vi "test_DataCollectionDL090215.vi"() -> ()   [LabVIEW 2010, in "DataCollectionDL090215.lvclass"]
uses:
  DataCollectionDL090215.lvclass
  common/classes/Image/Image/Image.lvclass
  main/labview_source/type_definitions/clusters/controls_refs.ctl
  common/classes/ErrorController/ErrorController/ErrorController.lvclass
  GenericDataCollection/GenericDataCollection/trigger_enum.ctl
  GenericDataCollection/GenericDataCollection/GenericDataCollection.lvclass
  common/classes/GenericToplevelComponent/GenericToplevelComponent/common_trigger_enum.ctl
  common/classes/GenericToplevelComponent/GenericToplevelComponent/GenericToplevelComponent.lvclass
panel:
  in  "images per sweep":i32
  in  "create":bool
  in  "reset":bool
  in  "save":bool
  out "event handling loop counter":i32=5
  in  "image index":i32
  in  "sweep index":i32
  in  "update":bool
  in  "retrieve":bool
  in  "insert":bool
  in  "stop":bool
  # "Test DL090215DataCollection"
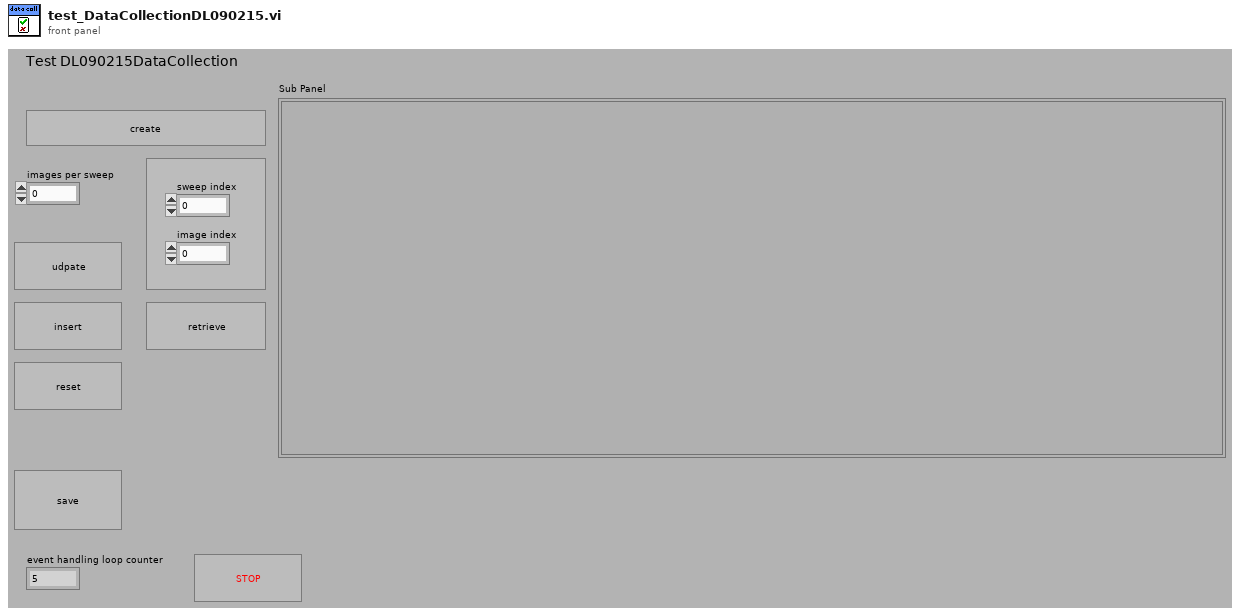
[diagram p1: front panel]
types:
  T1 = typedef "controls_refs.ctl" = cluster{"scan start button":refnum<vi>, "tabs":cluster{"main":refnum<vi>, "settings":refnum<vi>}, "subpanels":cluster{"imagingMode":refnum<vi>, "scanHead":refnum<vi>, "display":refnum<vi>, "experimentController":refnum<vi>, "instrument":refnum<vi>, "stage":refnum<vi>, "stimulator":refnum<vi>, "dataCollection":refnum<vi>, "analyser":refnum<vi>, "daq":refnum<vi>, "imageAssembler":refnum<vi>}, "drop-downs":cluster{"run mode":refnum<vi>, "imagingMode":refnum<vi>, "experimentalController":refnum<vi>, "objective":refnum<vi>}, "status lights":cluster{"experimentController":refnum<vi>, "imagingMode":refnum<vi>, "scanHead":refnum<vi>, "daq":refnum<vi>, "imageAssembler":refnum<vi>, "dataCollection":refnum<vi>, "display":refnum<vi>, "analyser":refnum<vi>, "stage":refnum<vi>, "stimulator":refnum<vi>, "instrument":refnum<vi>}, "message":refnum<vi>, "stimulator enabled?":refnum<vi>, "saving":cluster{"data folder path":refnum<vi>, "file base name":refnum<vi>, "notebook":refnum<vi>}, "progress bar":refnum<vi>, "update icon":refnum<vi>, "title":refnum<vi>, "main vi":refnum<vi>, "user":refnum<vi>, "exit_button":refnum<vi>, "CPU usage %":refnum<vi>}
  T2 = typedef "GenericDataCollection.lvclass/trigger_enum.ctl" = enum16{"NULL", "save"}
  T3 = typedef "GenericToplevelComponent.lvclass/common_trigger_enum.ctl" = enum16{"NULL", "initialise", "terminate", "fetch command", "fetch data", "attach observer", "register as observer", "detach observer", "acknowledge", "start", "stop"}
  T4 = typedef "Image Type" = u32
  T5 = typedef "plugin_specification.ctl" = cluster{"class path":string, "configuration":string, "label":string, "settings name":string}
  T6 = typedef "XComponentSpecification.xctl/data.ctl" = cluster{"class path":string, "configuration":string, "label":string, "settings name":string}
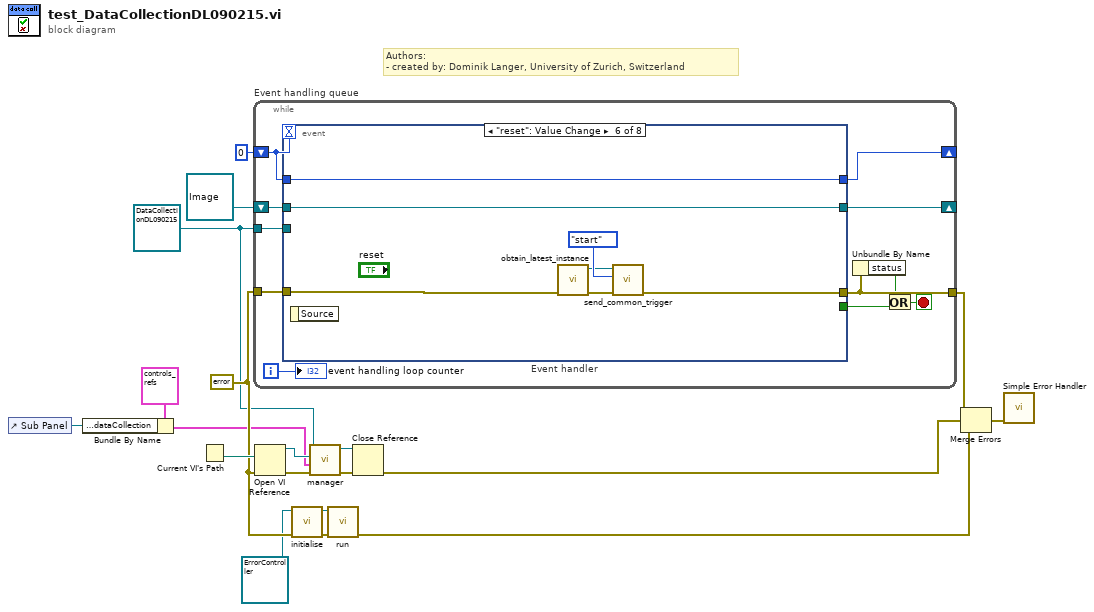
[diagram p0: block diagram]
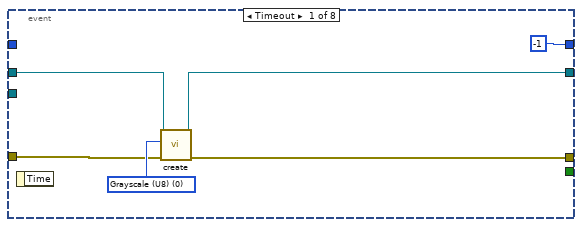
[diagram p2: hidden frame]
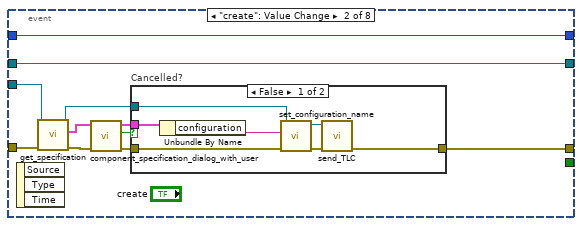
[diagram p3: hidden frame]
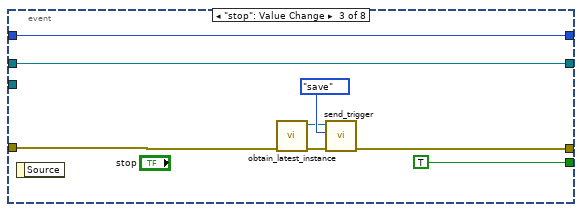
[diagram p5: hidden frame]
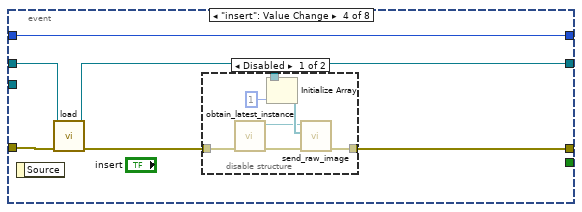
[diagram p6: hidden frame]
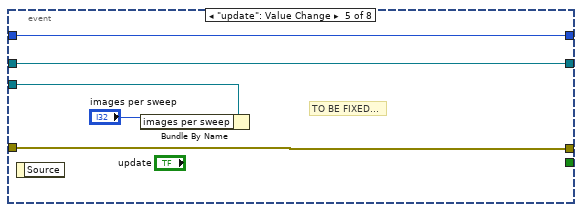
[diagram p8: hidden frame]
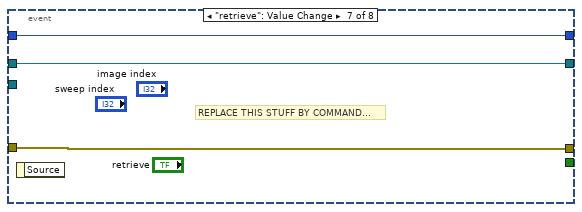
[diagram p9: hidden frame]
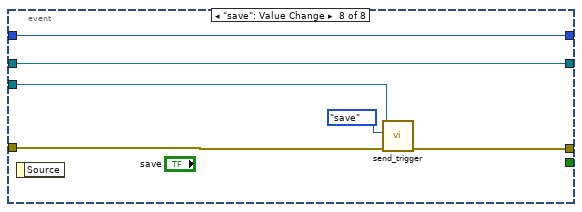
[diagram p10: hidden frame]
diagram:
  w1 = refnum<class "DataCollectionDL090215.lvclass"> refnum ("DL090215DataCollection.lvclass")
  w11 = errorcluster {"status"=FALSE, "code"=0, "source"=""} ("error out")
  # "Authors: \n- created by: Dominik Langer, University of Zurich, Switzerland"
  n1 = control-ref of="Sub Panel"() -> (w13:refnum<vi>)
  n2 = Bundle By Name(cluster=T1 {"scan start button"=refnum, "tabs"={"main"=refnum, "settings"=refnum}, "subpanels"={"imagingMode"=refnum, "scanHead"=refnum, "display"=refnum, "experimentController"=refnum, "instrument"=refnum, "stage"=refnum, "stimulator"=refnum, "dataCollection"=refnum, "analyser"=refnum, "daq"=refnum, "imageAssembler"=refnum}, "drop-downs"={"run mode"=refnum, "imagingMode"=refnum, "experimentalController"=refnum, "objective"=refnum}, "status lights"={"experimentController"=refnum, "imagingMode"=refnum, "scanHead"=refnum, "daq"=refnum, "imageAssembler"=refnum, "dataCollection"=refnum, "display"=refnum, "analyser"=refnum, "stage"=refnum, "stimulator"=refnum, "instrument"=refnum}, "message"=refnum, "stimulator enabled?"=refnum, "saving"={"data folder path"=refnum, "file base name"=refnum, "notebook"=refnum}, "progress bar"=refnum, "update icon"=refnum, "title"=refnum, "main vi"=refnum, "user"=refnum, "exit_button"=refnum, "CPU usage %"=refnum} ("control references"), "subpanels.dataCollection"=w13) -> (w2:T1)
  n3 = Current VI's Path() -> (path=w15:path)
  n4 = while "Event handling queue" {
    shift-right: [w29] -> _
    shift-left: 0 -> [w30]
    shift-right: [w26] -> _
    shift-left: refnum<class "Image.lvclass"> refnum ("Image.lvclass") -> [w27]
    tunnel: w1 -> [w24]
    tunnel: w11 -> [w28]
    tunnel: [w23] -> w18
    i -> [w25]
    stop <- w20 stop-if-true
    n5 = event "Event handler" shown="[5] \"reset\": Value Change" {
      selector: _ -> [_ _ _ _ _ _ _ _]
      dyn-events: _ -> [_ _ _ _ _ _ _ _]
      timeout: w30 -> [_ _ _ _ _ _ _ _]
      tunnel: w30 -> [_ w47 w63 w69 w81 w88 w91 w97]
      tunnel: [-1 w47 w63 w69 w81 w88 w91 w97] -> w29
      tunnel: w28 -> [w31 w43 w56 w68 w77 w82 w89 w95]
      tunnel: [w32 w45 w60 w66 w77 w86 w89 w94] -> w23
      tunnel: [_ _ TRUE _ _ _ _ _] -> w22
      tunnel: w27 -> [w33 w46 w61 w67 w80 w87 w90 w92]
      tunnel: [w35 w46 w61 w65 w80 w87 w90 w92] -> w26
      tunnel: w24 -> [_ w44 _ _ w79 _ _ w93]
      event Timeout {
        w34 = T4 0 items=["Grayscale (U8)", "Grayscale (I16)", "Grayscale (SGL)", "Complex (CSG)", "RGB (U32)", "HSL (U32)", "RGB (U64)", "Grayscale (U16)"] ("Image Type")
        n6 = event-data() -> ()  [unwired: 2 out]
        n7 = call "create.vi"("error in (no error)"=w31, "Image Type"=w34, "Image in"=w33) -> ("error out"=w32:errorcluster, "Image out"=w35:refnum<class "Image.lvclass">)  [unwired: 1 in, 6 out]
      }
      event "create": Value Change {
        n8 = event-data() -> ()  [unwired: 4 out]
        n9 = call-dynamic "get_specification.vi"("error in (no error)"=w43, "GenericPlugin in"=w44) -> ("error out"=w41:errorcluster, "component specification"=w42:T5, "GenericPlugin out"=w39:refnum<class "DataCollectionDL090215.lvclass">)  [unwired: 6 in, 1 out]
        n10 = call "component_specification_dialog_with_user.vi"("error in (no error)"=w41, "component specification in"=w42) -> ("error out"=w40:errorcluster, "cancelled?"=w38:bool, "component specification out"=w37:T6)  [unwired: 7 in]
        n11 = case "Cancelled?" shown="False" w38 {
          tunnel: [w54 w55] -> w45
          tunnel: w40 -> [w51 w55]
          tunnel: w39 -> [w50 _]
          tunnel: w37 -> [w49 _]
          frame False {
            n12 = Unbundle By Name(w49) -> ("configuration"=w48:string)
            n13 = call-dynamic "set_configuration_name.vi"("error in (no error)"=w51, "configuration"=w48, "GenericPlugin.lvclass in"=w50) -> ("error out"=w53:errorcluster, "GenericPlugin.lvclass out"=w52:refnum<class "DataCollectionDL090215.lvclass">)  [unwired: 7 out]
            n14 = call-dynamic "send_TLC.vi"("error in (no error)"=w53, "GenericToplevelComponent in"=w52) -> ("error out"=w54:errorcluster)  [unwired: 8 in, 1 out]
          }
          frame True {
          }
        }
      }
      event "stop": Value Change {
        n15 = event-data() -> ()  [unwired: 2 out]
        n16 = call "obtain_latest_instance.vi"("error in (no error)"=w56) -> ("error out"=w57:errorcluster, "GenericDataCollection out"=w58:refnum<class "GenericDataCollection.lvclass">)  [unwired: 1 in, 8 out]
        n17 = call-dynamic "send_trigger.vi"("error in (no error)"=w57, "trigger"=trigger_enum."save", "GenericDataCollection in"=w58) -> ("error out"=w60:errorcluster)  [unwired: 8 out]
      }
      event "insert": Value Change {
        n18 = event-data() -> ()  [unwired: 2 out]
        n19 = call-dynamic "load.vi"("error in (no error)"=w68, "Image in"=w67) -> ("error out"=w64:errorcluster, "Image out"=w65:refnum<class "Image.lvclass">)  [unwired: 2 in, 6 out]
        n20 = disable-structure shown="Disabled" {
          disable-tunnel: [w76 _] -> w66
          disable-tunnel: w65 -> [w75 _]
          disable-tunnel: w64 -> [w70 _]
          frame Disabled {
            n21 = call "obtain_latest_instance.vi"("error in (no error)"=w70) -> ("error out"=w71:errorcluster, "GenericDataCollection out"=w72:refnum<class "GenericDataCollection.lvclass">)  [unwired: 1 in, 8 out]
            n22 = Initialize Array(w75, 1 ("dimension size")) -> (w73:refnum<class "Image.lvclass">[])
            n23 = call-dynamic "send_raw_image.vi"("error in (no error)"=w71, "image"=w73, "GenericDataCollection in"=w72) -> ("error out"=w76:errorcluster)  [unwired: 6 in, 2 out]
          }
          frame Enabled {
          }
        }
      }
      event "update": Value Change {
        # "TO BE FIXED..."
        n24 = event-data() -> ()  [unwired: 2 out]
        n25 = Bundle By Name(cluster=w79, "images per sweep"="images per sweep") -> ()  [unwired: 1 out]
      }
      event "reset": Value Change {
        n26 = event-data() -> ()  [unwired: 2 out]
        n27 = call "obtain_latest_instance.vi"("error in (no error)"=w82) -> ("error out"=w84:errorcluster, "GenericDataCollection out"=w83:refnum<class "GenericDataCollection.lvclass">)  [unwired: 1 in, 8 out]
        n28 = call-dynamic "send_common_trigger.vi"("error in (no error)"=w84, "trigger"=common_trigger_enum."start", "GenericToplevelComponent in"=w83) -> ("error out"=w86:errorcluster)  [unwired: 6 in, 2 out]
      }
      event "retrieve": Value Change {
        # "REPLACE THIS STUFF BY COMMAND..."
        n29 = event-data() -> ()  [unwired: 2 out]
      }
      event "save": Value Change {
        n30 = event-data() -> ()  [unwired: 2 out]
        n31 = call-dynamic "send_trigger.vi"("error in (no error)"=w95, "trigger"=trigger_enum."save", "GenericDataCollection in"=w93) -> ("error out"=w94:errorcluster)  [unwired: 8 out]
      }
    }
    n32 = Unbundle By Name(w23) -> ("status"=w21:bool)
    n33 = Or(x=w21, y=w22) -> (x .or. y?=w20:bool)
    "event handling loop counter" <- w25
  }
  n34 = Open VI Reference(vi path=w15, error in (no error)=w11) -> (vi reference=w3:refnum<vi>, error out=w6:errorcluster)  [unwired: 4 in]
  n35 = call-dynamic "initialise.vi"("error in (no error)"=w11, "ErrorController in"=refnum<class "ErrorController.lvclass"> refnum) -> ("error out"=w10:errorcluster, "ErrorController out"=w9:refnum<class "ErrorController.lvclass">)  [unwired: 8 in]
  n36 = call-dynamic "manager.vi"("error in (no error)"=w6, "control references"=w2, "top-level VI ref in"=w3, "GenericToplevelComponent in"=w1) -> ("error out"=w5:errorcluster, "top-level VI ref out"=w4:refnum<vi>)  [unwired: 5 in, 1 out]
  n37 = call "run.vi"("error in (no error)"=w10, "ErrorController in"=w9) -> ("error out"=w8:errorcluster)  [unwired: 8 in, 1 out]
  n38 = Close Reference(reference=w4, error in (no error)=w5) -> (error out=w14:errorcluster)
  n39 = Merge Errors(w18, w14, w8) -> (w17:errorcluster)
  n40 = call <vilib>:"Simple Error Handler.vi"("error in (no error)"=w17) -> ()  [unwired: 1 in, 8 out]
